vi "Ball Goal Post Velocity After Collision Calcul.vi"(9 "Movable in":refnum<class "Movable.lvclass">, 10 "Goal post in":refnum<class "Goal Post.lvclass">) -> (1 "Movable out":refnum<class "Movable.lvclass">)   [LabVIEW 2024, in "Game Board.lvclass"]
doc: "MIT Licence\nCopyright (c) 2024 David Grollier"
uses:
  Game Board.lvclass
  Game Board Component/Movable/Movable.lvclass
  Game Board Component/Fixed/Board/Goal post/Goal Post.lvclass
  Type Def/Velocity.ctl
  Game Board Component/Movable/Movable.lvclass/Movable.ctl
  Game Componants.lvclass/Game Componants.ctl
  Game Componants.lvclass
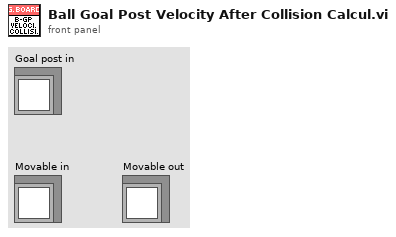
[diagram p1: front panel]
types:
  T1 = typedef "Velocity.ctl" = cluster{"Vx":dbl, "Vy":dbl}
  T2 = typedef "Coordinates.ctl" = cluster{"x":dbl, "y":dbl}
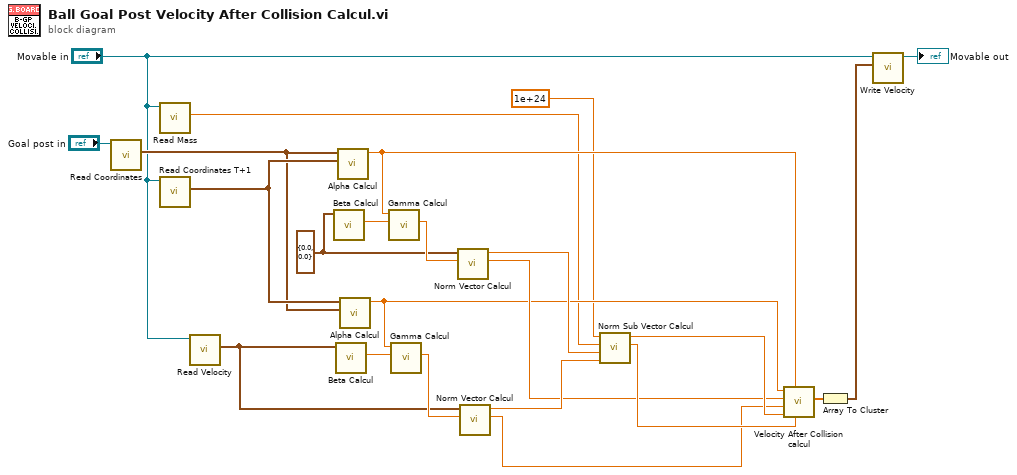
[diagram p0: block diagram]
diagram:
  w3 = T1 {"Vx"=0.0, "Vy"=0.0} ("Velocity")
  n1 = call "Read Coordinates.vi"("Game Componants in"="Goal post in") -> ("Coordinates"=w4:T2)  [unwired: 10 in]
  n2 = call "Read Mass.vi"("Movable in"="Movable in") -> ("Mass"=w10:dbl)  [unwired: 10 in]
  n3 = call "Read Coordinates T+1.vi"("Movable in"="Movable in") -> ("Coordinates"=w7:T2)  [unwired: 10 in]
  n4 = call-dynamic "Read Velocity.vi"("Movable in"="Movable in") -> ("Velocity"=w9:T1)  [unwired: 10 in]
  n5 = call "Beta Calcul.vi"("Velocity in"=w3) -> ("Beta out"=w22:dbl)  [unwired: 10 in]
  n6 = call "Beta Calcul.vi"("Velocity in"=w9) -> ("Beta out"=w19:dbl)  [unwired: 10 in]
  n7 = call "Alpha Calcul.vi"("Coordinates 2 in"=w7, "Coordinates 1 in"=w4) -> ("Alpha out"=w13:dbl)  [unwired: 9 in]
  n8 = call "Alpha Calcul.vi"("Coordinates 2 in"=w4, "Coordinates 1 in"=w7) -> ("Alpha out"=w12:dbl)  [unwired: 9 in]
  n9 = call "Gamma Calcul.vi"("Beta in"=w22, "Alpha in"=w13) -> ("Gamma out"=w21:dbl)  [unwired: 9 in]
  n10 = call "Gamma Calcul.vi"("Beta in"=w19, "Alpha in"=w12) -> ("Gamma out"=w20:dbl)  [unwired: 9 in]
  n11 = call "Norm Vector Calcul.vi"("Gamma"=w21, "Velocity in"=w3) -> ("Vector u11/22"=w14:dbl, "Vector u21/12"=w17:dbl)  [unwired: 8 in]
  n12 = call "Norm Vector Calcul.vi"("Gamma"=w20, "Velocity in"=w9) -> ("Vector u11/22"=w15:dbl, "Vector u21/12"=w18:dbl)  [unwired: 8 in]
  n13 = call "Norm Sub Vector Calcul.vi"("u21"=w18, "u12"=w17, "m2"=w10, "m1"=1e+24) -> ("v21"=w23:dbl, "v12"=w16:dbl)  [unwired: 6 in]
  n14 = call "Velocity After Collision calcul.vi"("v21"=w23, "Alpha1 in"=w13, "v12"=w16, "u22"=w15, "u11"=w14, "Alpha2 in"=w12) -> ("V2 out"=w11:dbl[])  [unwired: 4 in, 1 out]
  n15 = Array To Cluster(array=w11) -> (cluster=w8:cluster{"V2 out[0]":dbl, "V2 out[1]":dbl})
  n16 = call "Write Velocity.vi"("Velocity"=w8, "Movable in"="Movable in") -> ("Movable out"=→"Movable out":refnum<class "Movable.lvclass">)  [unwired: 9 in]
